vi "Test.vi"() -> ()   [LabVIEW 2021]
uses:
  Globals/Global message.vi
  Globals/CH1.vi
panel:
  in  "stop":bool
  in  "String":string
  in  "Numeric":dbl
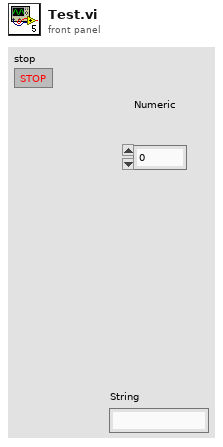
[diagram p1: front panel]
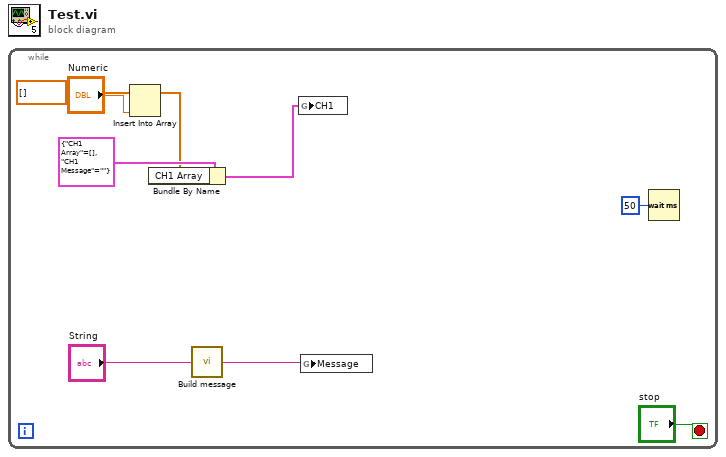
[diagram p0: block diagram]
diagram:
  n1 = while {
    stop <- "stop" stop-if-true
    n2 = Insert Into Array(array=dbl[] [], new element="Numeric") -> (w5:dbl[])  [unwired: 1 in]
    n3 = Bundle By Name(cluster=cluster{"CH1 Array":dbl[], "CH1 Message":string} {"CH1 Array"=[], "CH1 Message"=""} ("CH1"), "CH1 Array"=w5) -> (w4:cluster{"CH1 Array":dbl[], "CH1 Message":string})
    n4 = call "Build message.vi"("Input string"="String") -> ("Output string"=w1:string)
    n5 = global write "CH1.vi" "CH1"(w4) -> ()
    n6 = global write "Global message.vi" "Message"(w1) -> ()
    n7 = Wait (ms)(milliseconds to wait=u32 50) -> ()  [unwired: 1 out]
  }
